vi "Inverse Kinematics.vi"(11 "p":dbl[](array[numeric])) -> (2 "exist":bool, 3 "joints":dbl[](array[numeric]))   [LabVIEW 2013]
uses:
  <vilib>/Analysis/baseanly.llb/A x Vector.vi
  <vilib>/Analysis/_algsub.llb/Vector Norm.vi
  <vilib>/Analysis/_algsub.llb/Real Vector Norm.vi
  <vilib>/Analysis/baseanly.llb/Outer Product.vi
  <vilib>/Analysis/baseanly.llb/Real Outer Product.vi
  <vilib>/robotics/Kinematics/Create Lie Group Matrix.vi
  <vilib>/Analysis/7linalg.llb/Create Special Matrix.vi
  <vilib>/Analysis/7linalg.llb/Create Special Real Matrix.vi
  <vilib>/Analysis/Matrix/Numeric/Multiply/Multiply.vi
  <vilib>/Analysis/Matrix/Numeric/Multiply/Multiply - RM,R.vi
  <vilib>/Analysis/Matrix/Numeric/Multiply/Multiply - R,RM.vi
  <vilib>/Analysis/Matrix/Numeric/Add/Add.vi
  <vilib>/Analysis/Matrix/Numeric/Add/Add - RM,RM.vi
  Delta Robot Kinematics/Delta Robot Kinematics.lvclass
  <vilib>/robotics/Kinematics/NI_Kinematics.lvlib
  <vilib>/Analysis/NI_AALBase.lvlib
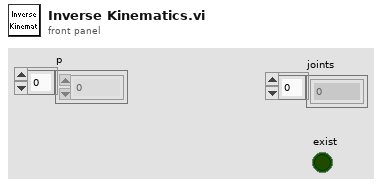
[diagram p1: front panel]
types:
  T1 = typedef "NI_Matrix.lvlib/RealMatrix.ctl" = dbl[][]
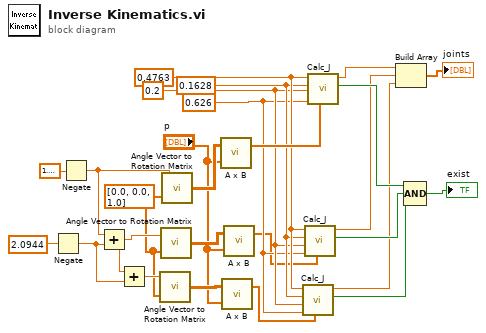
[diagram p0: block diagram]
diagram:
  w20 = dbl[] [0.0, 0.0, 1.0] ("vector")
  w15 = 0.626 ("re")
  w16 = 0.2 ("rf")
  w17 = 0.1628 ("e")
  w18 = 0.4763 ("f")
  n1 = Negate(x=2.0944 ("y")) -> (-x=w1:dbl)
  n2 = Negate(x=1.5707963267948966) -> (-x=w24:dbl)
  n3 = Add(x=w24, y=w1) -> (x+y=w21:dbl)
  n4 = Add(x=w21, y=w1) -> (x+y=w22:dbl)
  n5 = call <vilib>:"Angle Vector to Rotation Matrix.vi"("vector"=w20, "angle"=w22) -> ("rotation matrix"=w19:T1)
  n6 = call <vilib>:"Angle Vector to Rotation Matrix.vi"("vector"=w20, "angle"=w21) -> ("rotation matrix"=w23:T1)
  n7 = call <vilib>:"Angle Vector to Rotation Matrix.vi"("vector"=w20, "angle"=w24) -> ("rotation matrix"=w4:T1)
  n8 = call-poly <vilib>:"A x B.vi"("Vector"="p", "A"=w4) -> ("A x Vector"=w25:dbl[])  [unwired: 1 out]
  n9 = call-poly <vilib>:"A x B.vi"("Vector"="p", "A"=w19) -> ("A x Vector"=w13:dbl[])  [unwired: 1 out]
  n10 = call-poly <vilib>:"A x B.vi"("Vector"="p", "A"=w23) -> ("A x Vector"=w14:dbl[])  [unwired: 1 out]
  n11 = call "Calc_J.vi"("p"=w13, "re"=w15, "rf"=w16, "e"=w17, "f"=w18) -> ("exist"=w10:bool, "theta"=w6:dbl)  [unwired: 5 in]
  n12 = call "Calc_J.vi"("p"=w14, "re"=w15, "rf"=w16, "e"=w17, "f"=w18) -> ("exist"=w11:bool, "theta"=w7:dbl)  [unwired: 5 in]
  n13 = call "Calc_J.vi"("p"=w25, "re"=w15, "rf"=w16, "e"=w17, "f"=w18) -> ("exist"=w12:bool, "theta"=w8:dbl)  [unwired: 5 in]
  n14 = Build Array(w8, w7, w6) -> (→"joints":dbl[])
  n15 = Compound Arithmetic op=AND(w12, w11, w10) -> (→"exist":bool)
